vi "RandomInserting.vi"() -> ()   [LabVIEW 2019]
uses:
  <vilib>/addons/database/Auxilliary.llb/DB Tools Parameter Info.ctl
  <vilib>/addons/database/Auxilliary.llb/DB Tools DataTypes.ctl
  <vilib>/addons/database/Auxilliary.llb/DB Tools Parameter Dir.ctl
  <vilib>/addons/database/Connection.llb/DB Tools Open Connec (String).vi
  <vilib>/addons/database/Auxilliary.llb/DB Tools Format Datetime String (Time Stamp).vi
  <vilib>/addons/database/Command.llb/Cmd Set Parameter Value (C).vi
  <vilib>/addons/database/Command.llb/Cmd Execute.vi
  <vilib>/addons/database/Recordset.llb/Rec Destroy - Command.vi
  <vilib>/addons/database/NI_Database_API.lvlib
panel:
  in  "Time Stamp":timestamp
  out "current Length":dbl
  out "Current time stamp":timestamp
  out "No of Insertion In Db":i32
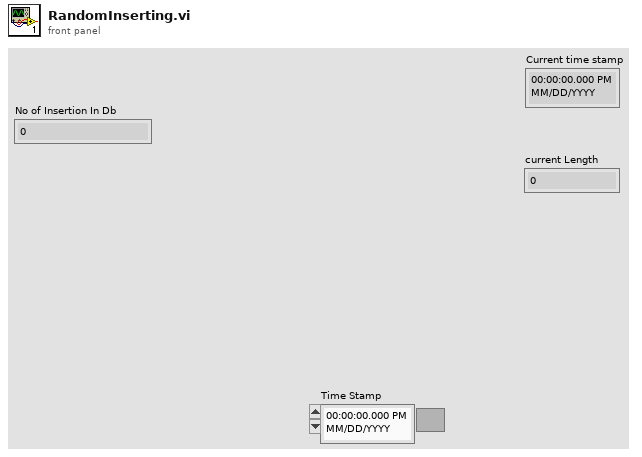
[diagram p1: front panel]
types:
  T1 = typedef "NI_Database_API.lvlib/Conn ObjectReference.ctl" = refnum<k1>
  T2 = typedef "NI_Database_API.lvlib/DB Tools Parameter Info.ctl" = cluster{"parameter name":string, "type":T3, "direction":T4, "value":variant}
  T3 = typedef "NI_Database_API.lvlib/DB Tools DataTypes.ctl" = enum16{"String", "Long (I32)", "Single (SGL)", "Double (DBL)", "Date/Time", "Binary"}
  T4 = typedef "NI_Database_API.lvlib/DB Tools Parameter Dir.ctl" = enum32{"Input", "Output", "Input/Output", "Return Value"}
  T5 = typedef "NI_Database_API.lvlib/Cmd ObjectReference.ctl" = refnum<k1>
  T6 = typedef "NI_Database_API.lvlib/Cmd-Rec Object Reference.ctl" = refnum<k1>
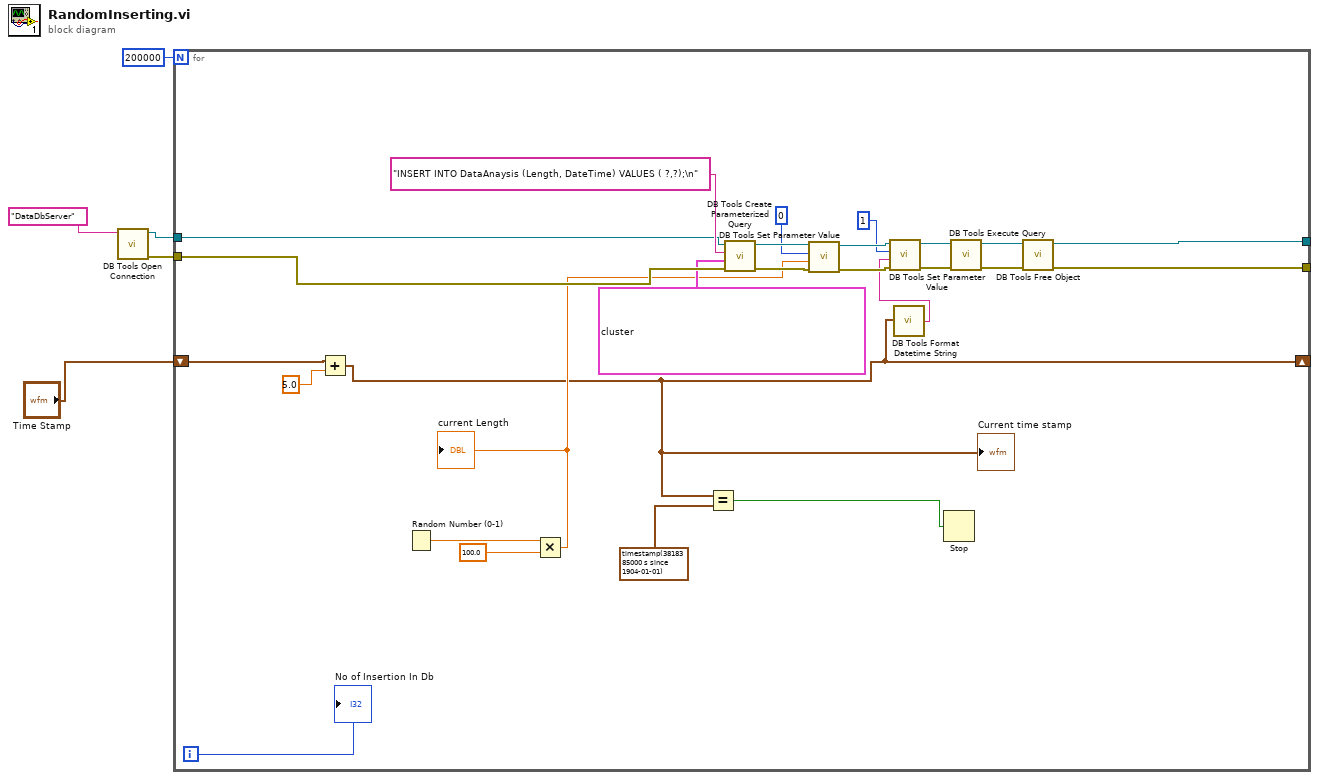
[diagram p0: block diagram]
diagram:
  n1 = call-poly <vilib>:"DB Tools Open Connection.vi"("connection information"="DataDbServer") -> ("error out"=w5:errorcluster, "connection reference"=w4:T1)  [unwired: 7 in]
  n2 = for {
    N: 200000 -> [_]
    shift-right: [w9] -> _
    shift-left: "Time Stamp" -> [w29]
    tunnel: w5 -> [w26]
    tunnel: w4 -> [w25]
    tunnel: [w11] -> _
    tunnel: [w10] -> _
    i -> [w7]
    n3 = Add(x=w29, y=5.0) -> (x+y=w9:timestamp)
    "Current time stamp" <- w9
    n4 = Random Number (0-1)() -> (number: 0 to 1=w30:dbl)
    n5 = Multiply(x=w30, y=100.0) -> (x*y=w20:dbl)
    "current Length" <- w20
    n6 = Equal?(x=w9, y=timestamp(3818385000 s since 1904-01-01)) -> (x = y?=w6:bool)
    n7 = call <vilib>:"DB Tools Create Parameterized Query.vi"("error in (no error)"=w26, "parameters"=T2[] [{"parameter name"="Length", "type"=enum."Double (DBL)", "direction"=enum."Input", "value"=variant}, {"parameter name"="DateTime", "type"=enum."Date/Time", "direction"=enum."Input", "value"=variant}], "SQL query"="INSERT INTO DataAnaysis (Length, DateTime) VALUES ( ?,?);\n", "connection reference"=w25) -> ("error out"=w22:errorcluster, "command reference"=w23:T5)  [unwired: 3 in, 1 out]
    n8 = call-poly <vilib>:"DB Tools Set Parameter Value.vi"("error in (no error)"=w22, "value"=w20, "parameter index"=0, "command reference"=w23) -> ("error out"=w19:errorcluster, "command reference out"=w18:T5)  [unwired: 4 in]
    n9 = call-poly <vilib>:"DB Tools Format Datetime String.vi"("time stamp"=w9) -> ("date/time string"=w14:string)
    n10 = call-poly <vilib>:"DB Tools Set Parameter Value.vi"("error in (no error)"=w19, "value"=w14, "parameter index"=1, "command reference"=w18) -> ("error out"=w16:errorcluster, "command reference out"=w15:T5)  [unwired: 4 in]
    n11 = Stop(stop? (T)=w6) -> ()
    n12 = call-poly <vilib>:"DB Tools Execute Query.vi"("error in (no error)"=w16, "command reference"=w15) -> ("error out"=w13:errorcluster, "command-recordset reference"=w12:T6)  [unwired: 6 in]
    n13 = call-poly <vilib>:"DB Tools Free Object.vi"("error in (no error)"=w13, "command-recordset reference"=w12) -> ("error out"=w10:errorcluster, "command reference"=w11:T5)  [unwired: 8 in]
    "No of Insertion In Db" <- w7
  }
